vi "Register gRPC Methods.vi"(8 "error in (no error)":errorcluster, 11 "Template Server in":refnum<class "veristand-grpc.lvclass">) -> (0 "error out":errorcluster, 3 "Template Server out":refnum<class "veristand-grpc.lvclass">)   [LabVIEW 2020, in "Veristandgrpc_server.lvlib" / "veristand-grpc.lvclass"]
uses:
  veristand-grpc.lvclass
  typeDefs/Server Internal UEs.ctl
  typeDefs/Server Internal Message.ctl
  typeDefs/Server gRPC UEs.ctl
  <vilib>/gRPC/LabVIEW gRPC Library/Server API/typeDefs/gRPCId Cluster.ctl
  <vilib>/gRPC/LabVIEW gRPC Library/Shared/grpcId.ctl
  veristand-grpc.lvclass/veristand-grpc.ctl
  <vilib>/gRPC/LabVIEW gRPC Library/grpc-lvsupport-release.lvlib
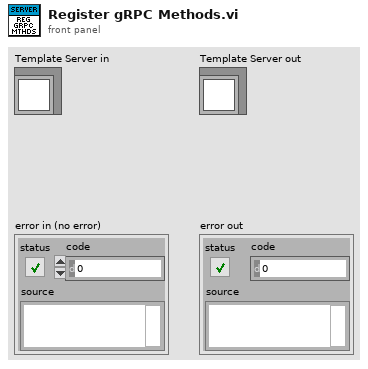
[diagram p1: front panel]
types:
  T1 = typedef "Veristandgrpc_server.lvlib/veristand-grpc.lvclass/Server gRPC UEs.ctl" = cluster{"veristand Write gRPC UE":refnum<user-event>, "veristand Read gRPC UE":refnum<user-event>}
  T2 = typedef "Veristandgrpc_server.lvlib/veristand-grpc.lvclass/Server Internal UEs.ctl" = cluster{"veristand Write Internal UE":refnum<user-event>, "veristand Read Internal UE":refnum<user-event>}
  T3 = typedef "grpc-lvsupport-release.lvlib/grpcId.ctl" = u64
  T4 = typedef "Veristandgrpc_server.lvlib/veristand-grpc.lvclass/Server Internal Message UE.ctl" = refnum<user-event>
  T5 = typedef "grpc-lvsupport-release.lvlib/gRPCId Cluster UE.ctl" = refnum<user-event>
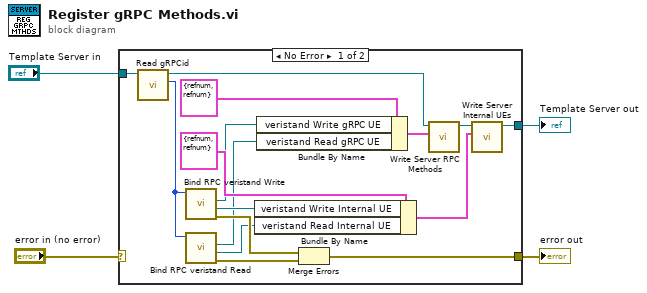
[diagram p0: block diagram]
diagram:
  n1 = case shown="No Error" "error in (no error)" {
    selector: "error in (no error)" -> [_ w21]
    tunnel: "Template Server in" -> [w12 w22]
    tunnel: [w20 w21] -> w3
    tunnel: [w19 w22] -> w2
    frame No Error {
      n2 = call-dynamic "Read gRPCid.vi"("iService in"=w12) -> ("gRPCid"=w11:T3, "iService out"=w13:refnum<class "veristand-grpc.lvclass">)  [unwired: 8 in, 1 out]
      n3 = call "Bind RPC veristand Write.vi"("gRPCid server in"=w11) -> ("error out"=w10:errorcluster, "veristand Write Internal UE"=w8:T4, "veristand Write gRPC UE"=w9:T5)  [unwired: 7 in, 1 out]
      n4 = call "Bind RPC veristand Read.vi"("gRPCid server in"=w11) -> ("error out"=w7:errorcluster, "veristand Read Internal UE"=w5:T4, "veristand Read gRPC UE"=w6:T5)  [unwired: 7 in, 1 out]
      n5 = Bundle By Name ("Bundle Internal UEs")(cluster=T2 {"veristand Write Internal UE"=refnum, "veristand Read Internal UE"=refnum} ("Server Internal UEs"), "veristand Write Internal UE"=w8, "veristand Read Internal UE"=w5) -> (w18:T2)
      n6 = Bundle By Name ("Bundle gRPC UEs")(cluster=T1 {"veristand Write gRPC UE"=refnum, "veristand Read gRPC UE"=refnum} ("gRPC Server Method Events"), "veristand Write gRPC UE"=w9, "veristand Read gRPC UE"=w6) -> (w15:T1)
      n7 = Merge Errors(w10, w7) -> (w20:errorcluster)
      n8 = call "Write Server RPC Methods.vi"("Server RPC Methods"=w15, "SignalGeneratorService in"=w13) -> ("SignalGeneratorService out"=w16:refnum<class "veristand-grpc.lvclass">)  [unwired: 8 in, 1 out]
      n9 = call "Write Server Internal UEs.vi"("Server Internal UEs"=w18, "SignalGeneratorService in"=w16) -> ("SignalGeneratorService out"=w19:refnum<class "veristand-grpc.lvclass">)  [unwired: 8 in, 1 out]
    }
    frame Error {
    }
  }
  "error out" <- w3
  "Template Server out" <- w2
